vi "ASDA-A2_Servo On(Off).vi"(8 "error in":errorcluster, 10 "On/Off":bool, 11 "Buffer Data In":T1) -> (0 "error out":errorcluster, 3 "Buffer Data Out":T1)   [LabVIEW 2016]
uses:
  Data Def/ASDA-A2_Buffer Data.ctl
  Data Def/ASDA-A2_Read Register Data.ctl
  Data Def/ASDA-A2_Write Register Data.ctl
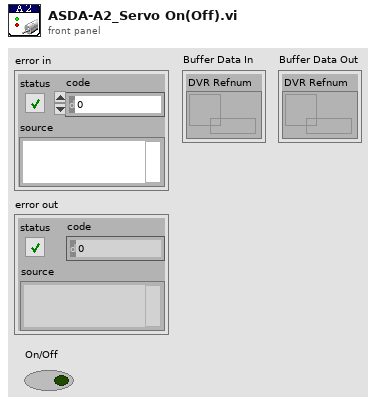
[diagram p1: front panel]
types:
  T1 = typedef "ASDA-A2_Buffer Data.ctl" = cluster{"DVR Refnum":refnum<data-value>}
  T2 = typedef "ASDA-A2_Write Register Data.ctl" = cluster{"Address":u16, "Max Value":u32, "Min Value":u32, "Value":u32, "Type":enum16{"16 Bits", "32 Bits"}, "Page":string, "Description":string}
  T3 = typedef "ASDA-A2_Read Register Data.ctl" = cluster{"Address":u16, "Count":u16, "Page":string, "Description":string}
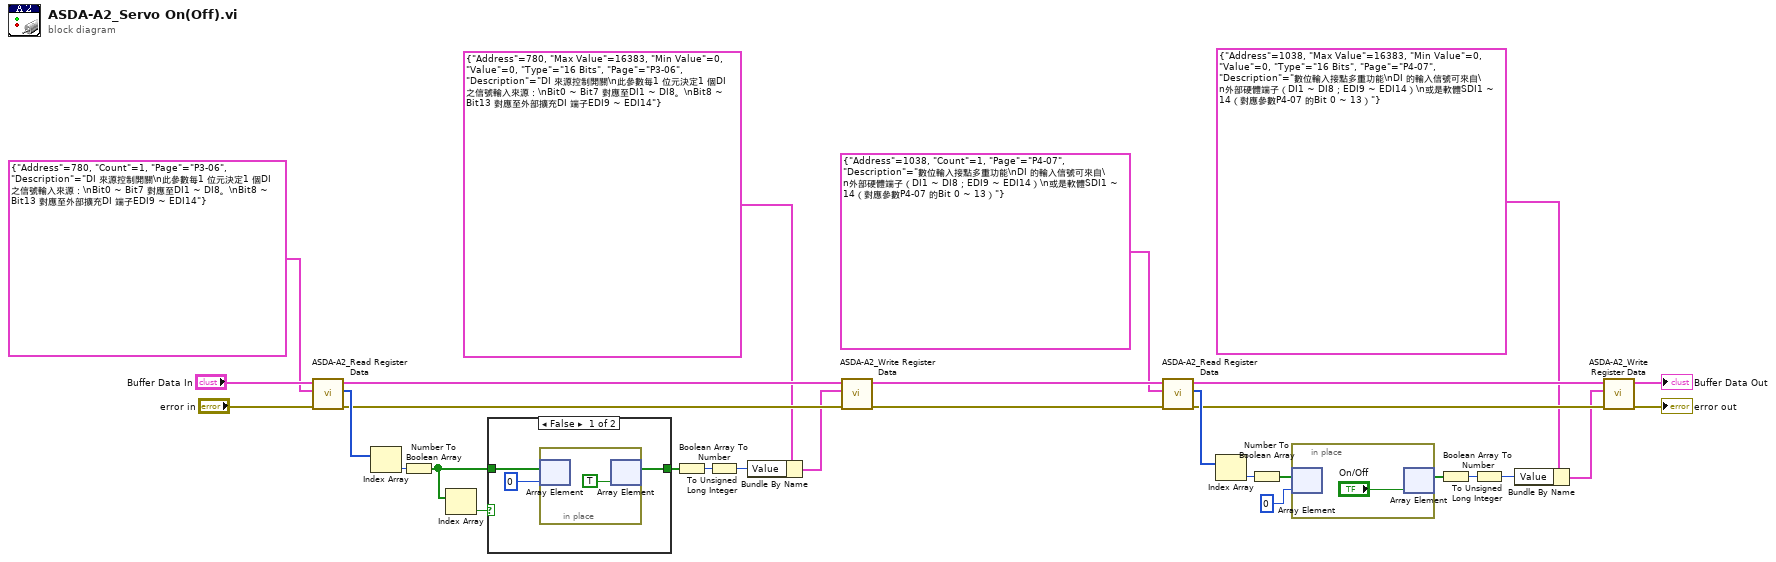
[diagram p0: block diagram]
diagram:
  n1 = call "ASDA-A2_Read Register Data.vi"("error in"="error in", "Read Register Data"=T3 {"Address"=780, "Count"=1, "Page"="P3-06", "Description"="DI 來源控制開關\n此參數每1 位元決定1 個DI 之信號輸入來源：\nBit0 ~ Bit7 對應至DI1 ~ DI8。\nBit8 ~ Bit13 對應至外部擴充DI 端子EDI9 ~ EDI14"}, "Buffer Data In"="Buffer Data In") -> ("error out"=w15:errorcluster, "Data"=w19:u16[], "Buffer Data Out"=w16:T1)  [unwired: 6 in]
  n2 = Index Array(array=w19) -> (element=w30:u16)  [unwired: 1 in]
  n3 = Number To Boolean Array(number=w30) -> (Boolean array=w23:bool[])
  n4 = Index Array(array=w23) -> (element=w24:bool)  [unwired: 1 in]
  n5 = case shown="False" w24 {
    tunnel: w23 -> [w33 w35]
    tunnel: [w31 w35] -> w17
    frame False {
      n6 = in-place {
        n7 = in-place-array #1(w33, 0) -> ()  [unwired: 1 out]
        n8 = in-place-array #1(TRUE ("element")) -> (w31:bool[])  [unwired: 1 out]
      }
    }
    frame True {
    }
  }
  n9 = Boolean Array To Number(Boolean array=w17) -> (number=w18:u32)
  n10 = To Unsigned Long Integer(number=w18) -> (unsigned 32bit integer=w13:u32)
  n11 = Bundle By Name(cluster=T2 {"Address"=780, "Max Value"=16383, "Min Value"=0, "Value"=0, "Type"=enum."16 Bits", "Page"="P3-06", "Description"="DI 來源控制開關\n此參數每1 位元決定1 個DI 之信號輸入來源：\nBit0 ~ Bit7 對應至DI1 ~ DI8。\nBit8 ~ Bit13 對應至外部擴充DI 端子EDI9 ~ EDI14"} ("Write Register Data"), "Value"=w13) -> (w12:T2)
  n12 = call "ASDA-A2_Write Register Data.vi"("error in"=w15, "Write Register Data"=w12, "Buffer Data In"=w16) -> ("error out"=w11:errorcluster, "Buffer Data Out"=w10:T1)  [unwired: 7 in]
  n13 = call "ASDA-A2_Read Register Data.vi"("error in"=w11, "Read Register Data"=T3 {"Address"=1038, "Count"=1, "Page"="P4-07", "Description"="數位輸入接點多重功能\nDI 的輸入信號可來自\n外部硬體端子（DI1 ~ DI8；EDI9 ~ EDI14）\n或是軟體SDI1 ~ 14（對應參數P4-07 的Bit 0 ~ 13）"}, "Buffer Data In"=w10) -> ("error out"=w6:errorcluster, "Data"=w8:u16[], "Buffer Data Out"=w7:T1)  [unwired: 6 in]
  n14 = Index Array(array=w8) -> (element=w25:u16)  [unwired: 1 in]
  n15 = Number To Boolean Array(number=w25) -> (Boolean array=w26:bool[])
  n16 = in-place {
    n17 = in-place-array #2(w26, 0) -> ()  [unwired: 1 out]
    n18 = in-place-array #2("On/Off") -> (w29:bool[])  [unwired: 1 out]
  }
  n19 = Boolean Array To Number(Boolean array=w29) -> (number=w28:u32)
  n20 = To Unsigned Long Integer(number=w28) -> (unsigned 32bit integer=w5:u32)
  n21 = Bundle By Name(cluster=T2 {"Address"=1038, "Max Value"=16383, "Min Value"=0, "Value"=0, "Type"=enum."16 Bits", "Page"="P4-07", "Description"="數位輸入接點多重功能\nDI 的輸入信號可來自\n外部硬體端子（DI1 ~ DI8；EDI9 ~ EDI14）\n或是軟體SDI1 ~ 14（對應參數P4-07 的Bit 0 ~ 13）"} ("Write Register Data"), "Value"=w5) -> (w3:T2)
  n22 = call "ASDA-A2_Write Register Data.vi"("error in"=w6, "Write Register Data"=w3, "Buffer Data In"=w7) -> ("error out"=→"error out":errorcluster, "Buffer Data Out"=→"Buffer Data Out":T1)  [unwired: 7 in]
